vi "Check Indices for Straight Continuous Line.vi"(11 "Letter Indices":T1[](array[typedef])) -> (3 "Straight Continuous Line?":bool)   [LabVIEW 2024, in "Wordle Scorer.lvlib"]
uses:
  Wordle Scorer.lvlib
  Letter Index--cluster.ctl
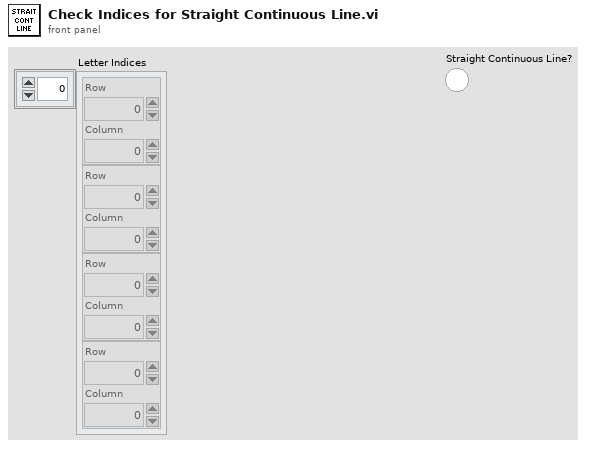
[diagram p1: front panel]
types:
  T1 = typedef "Wordle Scorer.lvlib/Letter Index--cluster.ctl" = cluster{"Row":i32, "Column":i32}
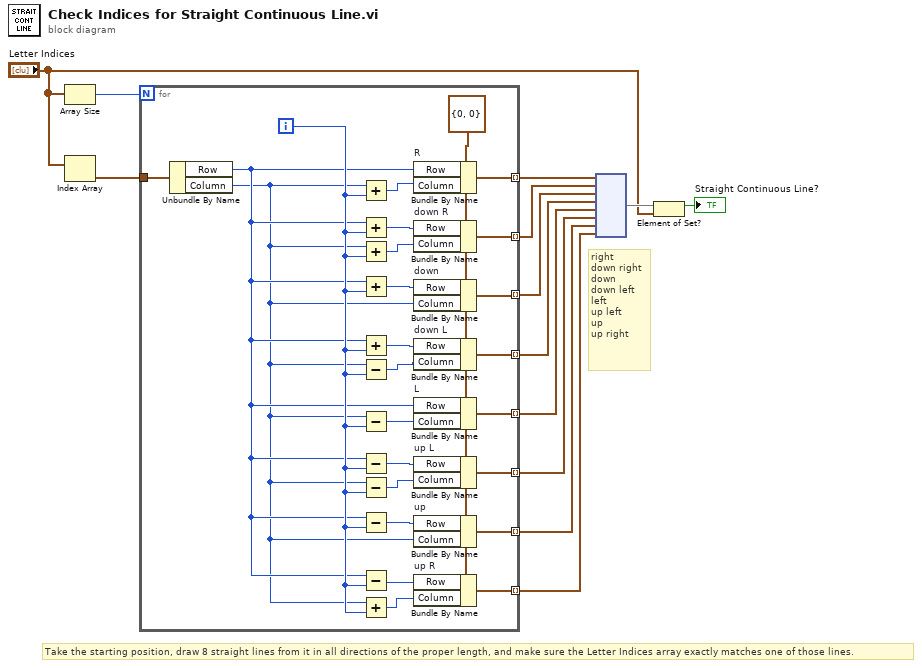
[diagram p0: block diagram]
diagram:
  # "Take the starting position, draw 8 straight lines from it in all directions of the proper length, and make sure the Letter Indices array exactly matches one of those lines."
  # "right\ndown right\ndown\ndown left\nleft\nup left\nup\nup right"
  n1 = Array Size(array="Letter Indices") -> (size(s)=w1:i32)
  n2 = Index Array(array="Letter Indices") -> (element=w13:T1)  [unwired: 1 in]
  n3 = for {
    N: w1 -> [_]
    tunnel: w13 -> [w29]
    tunnel: [w38] -> w12 mode=indexing
    tunnel: [w37] -> w11 mode=indexing
    tunnel: [w36] -> w10 mode=indexing
    tunnel: [w35] -> w9 mode=indexing
    tunnel: [w34] -> w8 mode=indexing
    tunnel: [w33] -> w7 mode=indexing
    tunnel: [w32] -> w6 mode=indexing
    tunnel: [w31] -> w5 mode=indexing
    i -> [w16]
    w30 = T1 {"Row"=0, "Column"=0} ("element")
    n4 = Unbundle By Name(w29) -> ("Row"=w15:i32, "Column"=w14:i32)
    n5 = Add(x=w14, y=w16) -> (x+y=w25:i32)
    n6 = Add(x=w15, y=w16) -> (x+y=w24:i32)
    n7 = Add(x=w14, y=w16) -> (x+y=w23:i32)
    n8 = Add(x=w15, y=w16) -> (x+y=w27:i32)
    n9 = Add(x=w15, y=w16) -> (x+y=w22:i32)
    n10 = Subtract(x=w14, y=w16) -> (x-y=w21:i32)
    n11 = Subtract(x=w14, y=w16) -> (x-y=w28:i32)
    n12 = Subtract(x=w15, y=w16) -> (x-y=w20:i32)
    n13 = Subtract(x=w14, y=w16) -> (x-y=w19:i32)
    n14 = Subtract(x=w15, y=w16) -> (x-y=w26:i32)
    n15 = Subtract(x=w15, y=w16) -> (x-y=w18:i32)
    n16 = Add(x=w14, y=w16) -> (x+y=w17:i32)
    n17 = Bundle By Name "R"(cluster=w30, "Row"=w15, "Column"=w25) -> (w38:T1)
    n18 = Bundle By Name "down R"(cluster=w30, "Row"=w24, "Column"=w23) -> (w37:T1)
    n19 = Bundle By Name "down"(cluster=w30, "Row"=w27, "Column"=w14) -> (w36:T1)
    n20 = Bundle By Name "down L"(cluster=w30, "Row"=w22, "Column"=w21) -> (w35:T1)
    n21 = Bundle By Name "L"(cluster=w30, "Row"=w15, "Column"=w28) -> (w34:T1)
    n22 = Bundle By Name "up L"(cluster=w30, "Row"=w20, "Column"=w19) -> (w33:T1)
    n23 = Bundle By Name "up"(cluster=w30, "Row"=w26, "Column"=w14) -> (w32:T1)
    n24 = Bundle By Name "up R"(cluster=w30, "Row"=w18, "Column"=w17) -> (w31:T1)
  }
  n25 = node(w12, w11, w10, w9, w8, w7, w6, w5) -> (w4:set{T1[]})
  n26 = Element of Set?(10:"Letter Indices", 11:w4) -> (3:→"Straight Continuous Line?":bool)
